vi "GetMaxMin.vi"(8 "error in (no error)":errorcluster, 10 "Ignore Cal? (F)":bool, 11 "Thermocouple in":refnum<class "Thermocouple.lvclass">) -> (0 "error out":errorcluster, 1 "Min":cluster{"Value":dbl, "Text":string}, 2 "Max":cluster{"Value":dbl, "Text":string}, 3 "Thermocouple out":refnum<class "Thermocouple.lvclass">)   [LabVIEW 2018, in "Measurement Channels.lvlib" / "Thermocouple.lvclass"]
uses:
  Thermocouple.lvclass
  C:/Users/Jeff Tipps/Documents/DAQMan/source/Classes/Measurements/Class Channel/Channel.lvclass
  Thermocouple.lvclass/Thermocouple.ctl
  Class Channel/Read Scale.vi
  Class Channel/Read Offset.vi
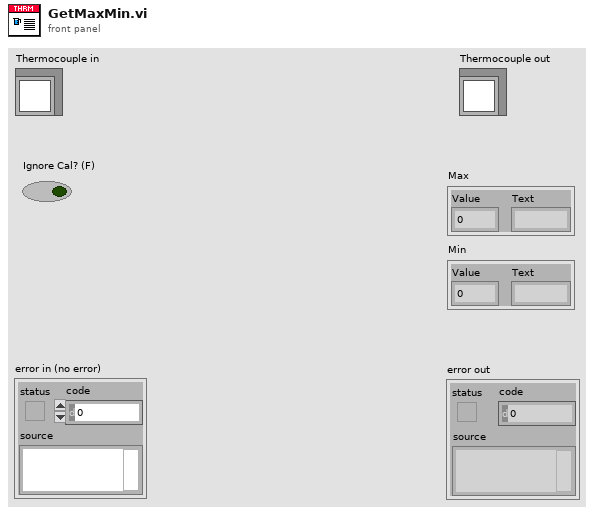
[diagram p1: front panel]
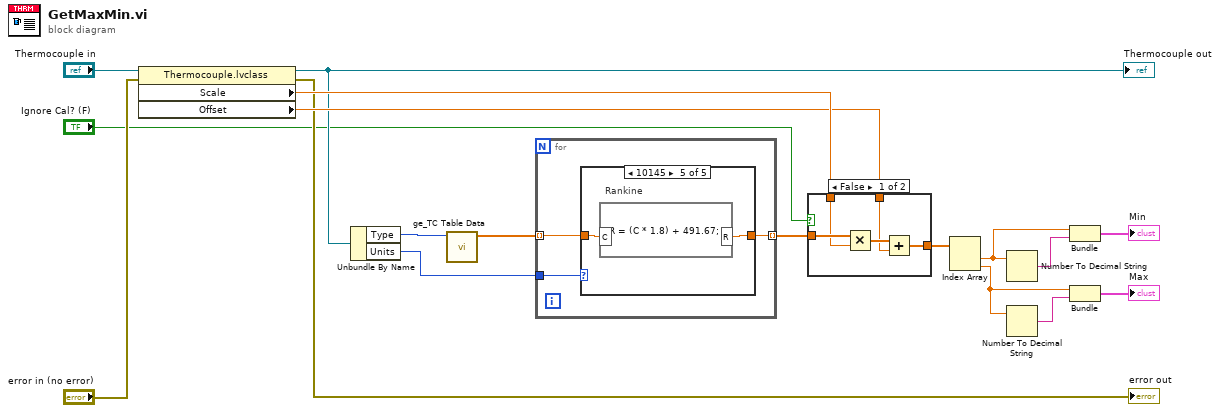
[diagram p0: block diagram]
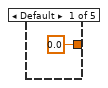
[diagram p3: hidden frame]
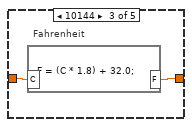
[diagram p5: hidden frame]
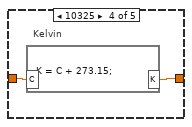
[diagram p6: hidden frame]
diagram:
  n1 = property class="Thermocouple.lvclass"(reference="Thermocouple in", error in="error in (no error)") -> (reference out=w10:refnum<class "Thermocouple.lvclass">, error out=→"error out":errorcluster, "Scale"=w12:dbl, "Offset"=w11:dbl)
  "Thermocouple out" <- w10
  n2 = Unbundle By Name(w10) -> ("Type"=w15:u16, "Units"=w14:u16)
  n3 = call "ge_TC Table Data.vi"("Thrmcpl Type"=w15) -> ("Type Min/Max"=w18:dbl[])  [unwired: 10 in]
  n4 = for {
    tunnel: w14 -> [w21]
    tunnel: [w20] -> w17 mode=indexing
    tunnel: w18 -> [w19] mode=indexing
    n5 = case shown="10145" w21 {
      tunnel: w19 -> [_ w23 w25 w27 w29]
      tunnel: [0.0 ("R") w23 w24 w26 w28] -> w20
      frame Default {
      }
      frame 10143 {
        # "Celsius"
      }
      frame 10144 {
        # "Fahrenheit"
        n6 = formula code="F = (C * 1.8) + 32.0;"("C"=w25) -> ("F"=w24:dbl)
      }
      frame 10325 {
        # "Kelvin"
        n7 = formula code="K = C + 273.15;"("C"=w27) -> ("K"=w26:dbl)
      }
      frame 10145 {
        # "Rankine"
        n8 = formula code="R = (C * 1.8) + 491.67;"("C"=w29) -> ("R"=w28:dbl)
      }
    }
  }
  n9 = case shown="False" "Ignore Cal? (F)" {
    tunnel: w17 -> [w34 w35]
    tunnel: [w32 w35] -> w16
    tunnel: w12 -> [w31 _]
    tunnel: w11 -> [w30 _]
    frame False {
      n10 = Multiply(x=w34, y=w31) -> (x*y=w33:dbl[])
      n11 = Add(x=w33, y=w30) -> (x+y=w32:dbl[])
    }
    frame True {
    }
  }
  n12 = Index Array(array=w16) -> (element #1=w7:dbl, element #2=w5:dbl)  [unwired: 2 in]
  n13 = Number To Decimal String(number=w7) -> (decimal integer string=w6:string)  [unwired: 1 in]
  n14 = Number To Decimal String(number=w5) -> (decimal integer string=w4:string)  [unwired: 1 in]
  n15 = Bundle("R"=w7, w6) -> (→"Min":cluster{"R":dbl, string})  [unwired: 1 in]
  n16 = Bundle("R"=w5, w4) -> (→"Max":cluster{"R":dbl, string})  [unwired: 1 in]
